vi "Speed Experiment -- JDP.vi"() -> ()   [LabVIEW 2011]
doc: "Demonstrates the use of the Variant JSON VIs for converting to and from a complex cluster."
uses:
  JSON Value/Set from JSON string.vi
  JSON Value/Get Array by name.vi
  JSON Scalar/Get as Text.vi
  JSON Value/JSON Value.lvclass
  Get Polymorphic/JSON GetSet.lvlib
  JSON Scalar/JSON Scalar.lvclass
panel:
  out "Time (s)":dbl format="%#_6p"
  in  "Application Config":string="{\"instruments\":[\"type\",\"SimMultimeter\",\"config\"],\n\"etc.\":\"...\"\n}"
  # "[{\"type\":\"SimMultimeter\",\"config\":{\"maxV\":10,\"maxI\",5}},\n{\"type\":\"SimVoltmeter\",\"config\": {\"maxV\":100}},\n{\"type\":\"SimDAQ\",\"config\": NULL}]"
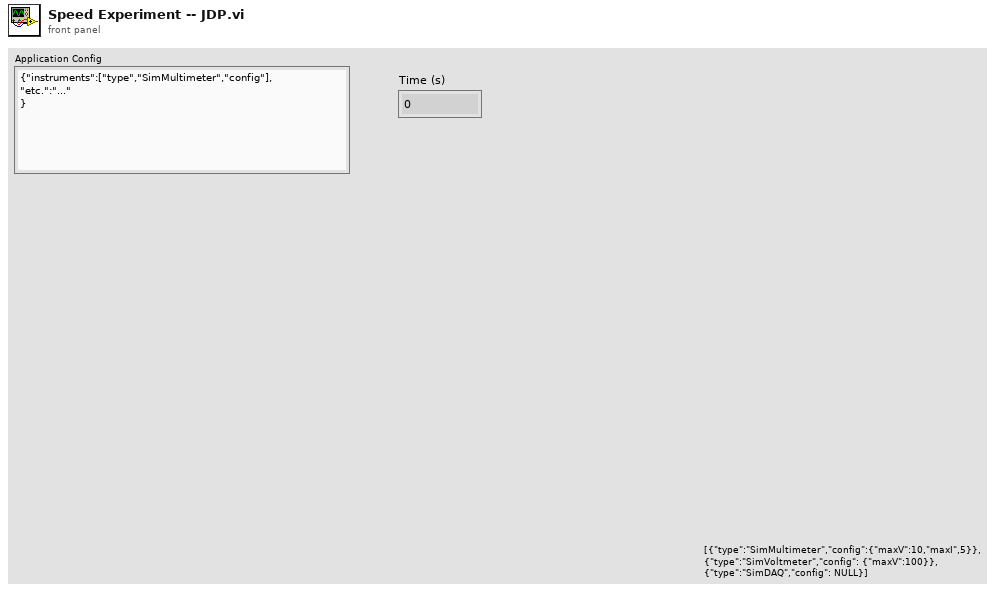
[diagram p1: front panel]
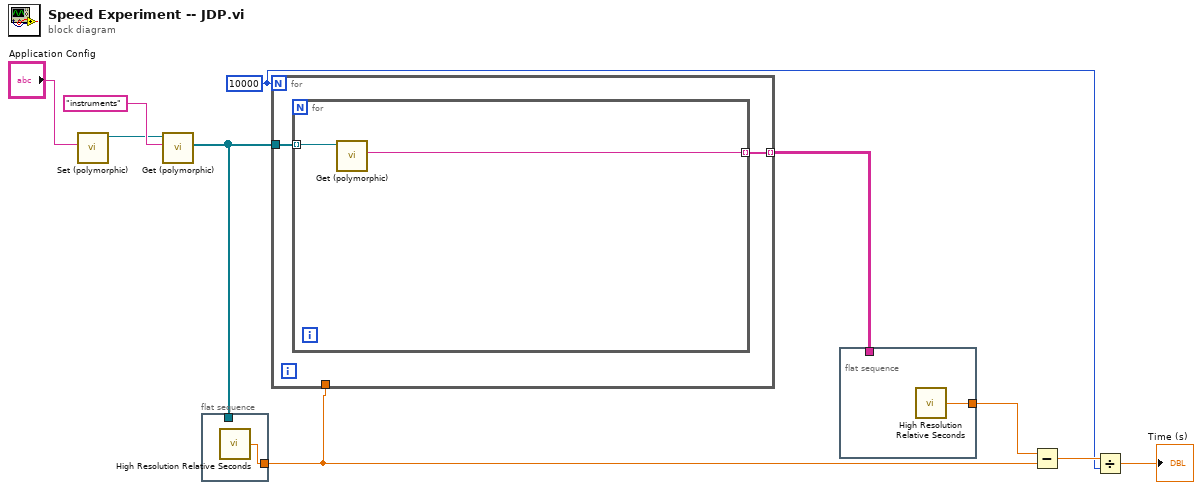
[diagram p0: block diagram]
diagram:
  w1 = 10000
  n1 = call-poly "Set (polymorphic).vi"("JSON stream"="Application Config") -> ("JSON Value out"=w8:refnum<class "JSON Value.lvclass">)  [unwired: 8 in, 2 out]
  n2 = call-poly "Get (polymorphic).vi"("name"="instruments", "JSON Value In"=w8) -> ("Array"=w4:refnum<class "JSON Value.lvclass">[])  [unwired: 6 in, 3 out]
  n3 = flat-sequence {
    tunnel: w4 -> [_]
    tunnel: [w11] -> w3
    frame #0 {
      n4 = call <vilib>:"High Resolution Relative Seconds.vi"() -> ("relative seconds"=w11:dbl)
    }
  }
  n5 = for {
    N: w1 -> [_]
    tunnel: w4 -> [w13]
    tunnel: [w12] -> w2 mode=indexing
    tunnel: w3 -> [_]
    n6 = for {
      tunnel: w13 -> [w15] mode=indexing
      tunnel: [w14] -> w12 mode=indexing
      n7 = call-poly "Get (polymorphic).vi"("JSON Scalar in"=w15) -> ("LabVIEW Text"=w14:string)  [unwired: 8 in, 2 out]
    }
  }
  n8 = flat-sequence {
    tunnel: [w16] -> w5
    tunnel: w2 -> [_]
    frame #0 {
      n9 = call <vilib>:"High Resolution Relative Seconds.vi"() -> ("relative seconds"=w16:dbl)
    }
  }
  n10 = Subtract(x=w5, y=w3) -> (x-y=w6:dbl)
  n11 = Divide(x=w6, y=w1) -> (x/y=→"Time (s)":dbl)
